vi "ReadChangedLibrariesLog.vi"(8 "error in (no error)":errorcluster) -> (0 "error out":errorcluster, 3 "ChangedLibraries":string[](array[string]))   [LabVIEW 2019, in "DepsWatch.lvlib"]
uses:
  DepsWatch.lvlib
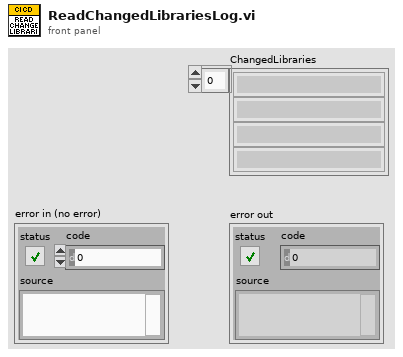
[diagram p1: front panel]
types:
  T1 = enum16{"open", "replace", "create", "open or create", "replace or create", "replace or create with confirmation"}
  T2 = typedef "DepsWatch.lvlib/CICDPathConfigs.ctl" = cluster{"GlobalIncludePaths":path[], "GlobalExcludePaths":path[], "BuildSpecsIncludePaths":path[], "ActualDepsIncludePaths":path[], "WorkspacePath":path, "SourceFolderPaths":path[], "ChangedFilesLogpaths":map{string, path}}
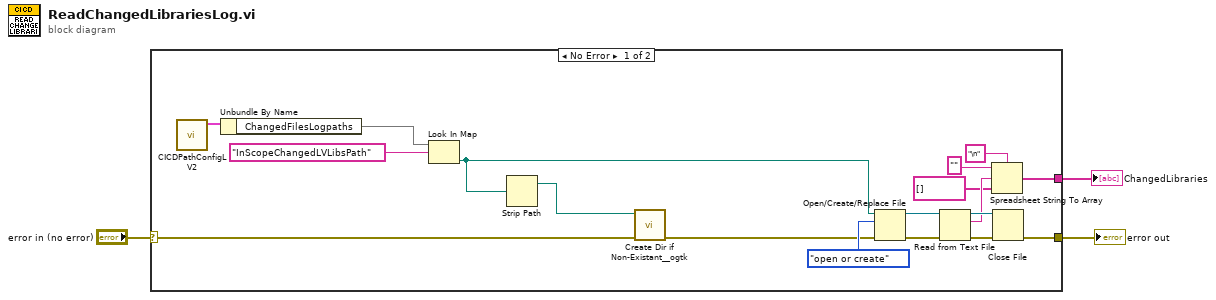
[diagram p0: block diagram]
diagram:
  n1 = case shown="No Error" "error in (no error)" {
    selector: "error in (no error)" -> [w5 w22]
    tunnel: [w9 _] -> w2
    tunnel: [w8 w22] -> w1
    frame No Error {
      n2 = call "CICDPathConfigLV2.vi"() -> ("CICD Path Config Out"=w21:T2)  [unwired: 11 in]
      n3 = Unbundle By Name(w21) -> ("ChangedFilesLogpaths"=w19:map{string, path})
      n4 = Look In Map(map=w19, key="InScopeChangedLVLibsPath") -> (value=w7:path)  [unwired: 1 in, 1 out]
      n5 = Strip Path(path=w7) -> (stripped path=w6:path)  [unwired: 1 out]
      n6 = call <userlib>:"Create Dir if Non-Existant__ogtk.vi"("error in (no error)"=w5, "Directory Path"=w6) -> ("error out"=w4:errorcluster)  [unwired: 7 in, 2 out]
      n7 = Open/Create/Replace File(file path (use dialog)=w7, error in=w4, operation (0:open)=T1."open or create") -> (refnum out=w17:refnum<file>, error out=w16:errorcluster)  [unwired: 3 in, 1 out]
      n8 = Read from Text File(file (use dialog)=w17, error in=w16) -> (refnum out=w15:refnum<file>, text=w13:string, error out=w14:errorcluster)  [unwired: 2 in, 1 out]
      n9 = Spreadsheet String To Array(delimiter (Tab)="\n", format string="", spreadsheet string=w13, array type (2D Dbl)=string[] []) -> (array=w9:string[])
      n10 = Close File(refnum=w15, error in=w14) -> (error out=w8:errorcluster)  [unwired: 1 out]
    }
    frame Error {
    }
  }
  "ChangedLibraries" <- w2
  "error out" <- w1
